vi "Shooter Controller.vi"(8 "error in":errorcluster) -> ()   [LabVIEW 2019]
doc: "This VI executes continuously carrying out the current operation and responding to updates or new operations. It will often contain the timing or control code that is difficult to place directly in TeleOp. This VI generally opens all sensors and motors and isolates the rest of the robot code from knowing how the operations are carried out."
uses:
  <vilib>/Rock Robotics/WPI/Framework/Completion Status.ctl
  Shooter Setpoints.ctl
  Shooter Operations.ctl
  <vilib>/Rock Robotics/WPI/MotorControl/WPI_MotorControlDeviceRef.ctl
  <vilib>/Rock Robotics/WPI/MotorControl/WPI_MotorControlType.ctl
  <vilib>/Rock Robotics/SystemInterfaces/DIO/FPGA_DIOPWMChannel.ctl
  <vilib>/Rock Robotics/WPI/PWM/WPI_PWMDeadband.ctl
  <vilib>/Rock Robotics/SystemInterfaces/DIO/FPGA_DIOChannel.ctl
  <vilib>/Rock Robotics/WPI/PWM/Servo/WPI_ServoDeviceRef.ctl
  <vilib>/Rock Robotics/WPI/ThirdParty/REV Robotics/SPARK MAX/Typedef/Spark MAX Motor Type.ctl
  <vilib>/Rock Robotics/WPI/ThirdParty/REV Robotics/SPARK MAX/Typedef/Spark MAX Control Type.ctl
panel:
  in  "Ramp Limit Rate (S)":sgl
  out "Shooter":T1(graph)
  in  "PID Shooter":T2={"P Gain"=0.00026, "I Gain"=0.0, "D Gain"=0.0, "F Gain"=0.0002, "I Zone"=0.0, "Min Output"=-1.0, "Max Output"=0.0} {"Max Output" min=-1.0 max=1.0 step=0.01; "Min Output" min=-1.0 max=1.0 step=0.01; "I Zone" step=0.01; "F Gain" step=0.01; "D Gain" step=0.01; "I Gain" step=0.01; "P Gain" min=0.0 step=0.01}
  in  "Interactive Values":T3
  out "Current\nCmd":string
  in  "Buttons":cluster{"Execute Cmd":bool, "Abort Cmd":bool}
  out "Command Timing":cluster{"Start Time (ms)":u32, "Iterations":i32}
  out "Status":T5
  # "Click here to set max"
  # "Click here to set min"
  # "Interactive Command: You may fill in the settings for a command\nand schedule it with the Execute button. You can observe and abort\nany command while fine tuning the code for the controller."
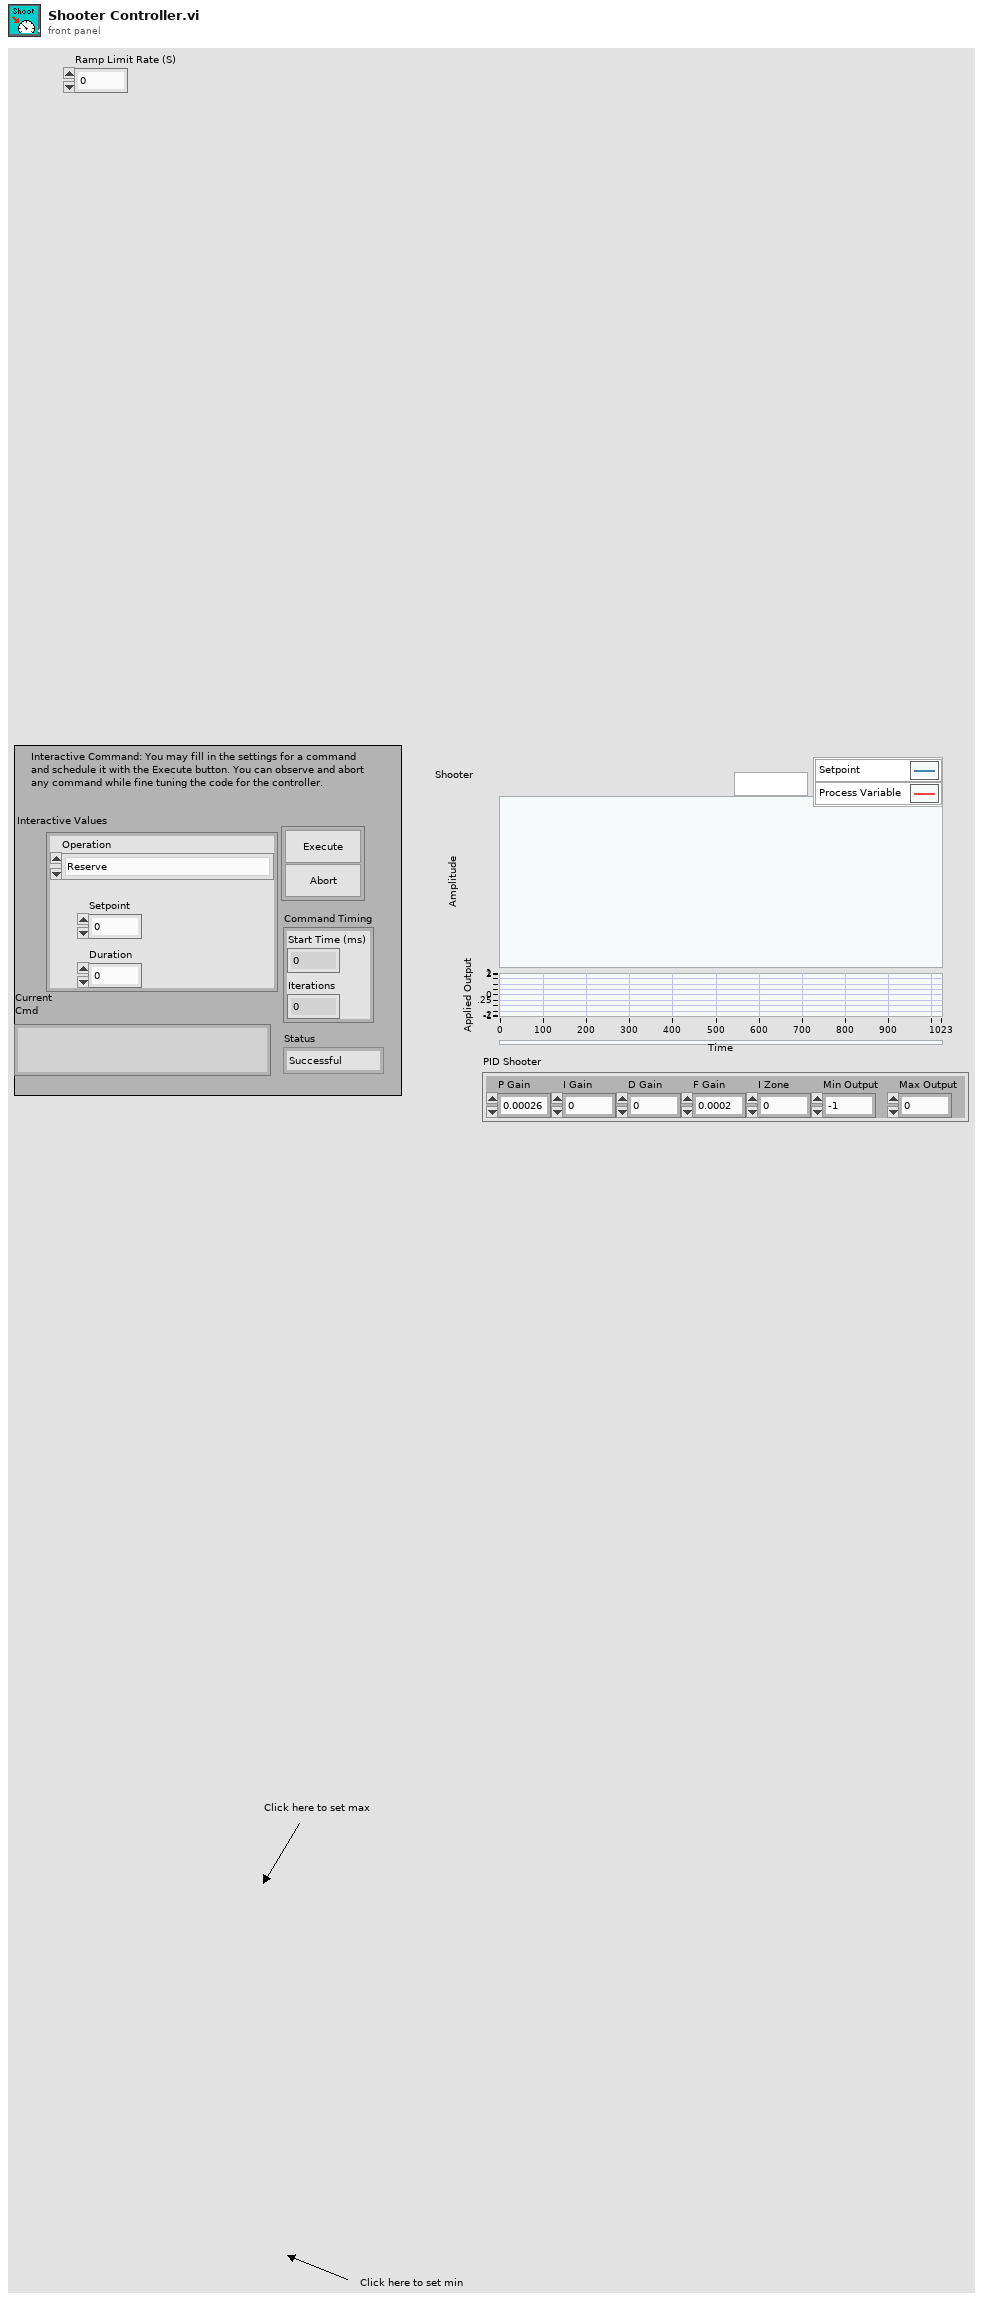
[diagram p1: front panel]
types:
  T1 = cluster{"Sensor Velocity":dbl, "Setpoint":dbl, "Applied Output":dbl}
  T2 = cluster{"P Gain":dbl, "I Gain":dbl, "D Gain":dbl, "F Gain":dbl, "I Zone":dbl, "Min Output":dbl, "Max Output":dbl}
  T3 = typedef "Shooter Setpoints.ctl" = cluster{"Operation":T4, "Setpoint":dbl, "Duration":dbl}
  T4 = typedef "Shooter Operations.ctl" = enum16{"Reserve", "Read Current", "Immediate", "Uptake", "Shooter", "Shift Winch", "Shift Uptake", "Shift Uptake Assist Up", "Shift Uptake Assist Down"}
  T5 = typedef "Completion Status.ctl" = enum16{"Successful", "Aborted", "Incomplete"}
  T6 = typedef "FPGA_DIOPWMChannel.ctl" = enum8{"PWM 0", "PWM 1", "PWM 2", "PWM 3", "PWM 4", "PWM 5", "PWM 6", "PWM 7", "PWM 8", "PWM 9", "PWM MXP 0", "PWM MXP 1", "PWM MXP 2", "PWM MXP 3", "PWM MXP 4", "PWM MXP 5", "PWM MXP 6", "PWM MXP 7", "PWM MXP 8", "PWM MXP 9", "Invalid"}
  T7 = typedef "Spark MAX Motor Type.ctl" = enum16{"Brushed", "Brushless"}
  T8 = typedef "WPI_MotorControlDeviceRef.ctl" = cluster{"DeviceStatus":errorcluster, "Type":T9, "PWM":cluster{"PWM Channel":T6, "DeadBand":T10}, "CAN":cluster{"Device Number":u8, "SetOutput VI Ref":variant, "GetOutput VI Ref":variant, "Enable VI Ref":variant, "Disable VI Ref":variant, "Data":variant}, "Invert":bool, "DIO PWM":cluster{"PWM \"Enable\" Channel":T6, "DIOChannel":T11, "PWM Rate":dbl}}
  T9 = typedef "WPI_MotorControlType.ctl" = enum16{"PWM", "CAN", "DIO PWM"}
  T10 = typedef "WPI_PWMDeadband.ctl" = cluster{"Name":string, "maxPositivePwm":i32, "minPositivePwm":i32, "centerPwm":i32, "maxNegativePwm":i32, "minNegativePwm":i32, "angularRange":u16}
  T11 = typedef "FPGA_DIOChannel.ctl" = enum8{"DIO 0", "DIO 1", "DIO 2", "DIO 3", "DIO 4", "DIO 5", "DIO 6", "DIO 7", "DIO 8", "DIO 9", "DIO MXP 0", "DIO MXP 1", "DIO MXP 2", "DIO MXP 3", "DIO MXP 4", "DIO MXP 5", "DIO MXP 6", "DIO MXP 7", "DIO MXP 8", "DIO MXP 9", "DIO MXP 10", "DIO MXP 11", "DIO MXP 12", "DIO MXP 13", "DIO MXP 14", "DIO MXP 15", "SPI Port CS1", "SPI Port CS2", "SPI Port CS3", "SPI Port MISO", "SPI Port MOSI", "Invalid"}
  T12 = typedef "WPI_ServoDeviceRef.ctl" = cluster{"DeviceStatus":errorcluster, "PWM Channel":T6, "DeadBand":T10}
  T13 = cluster{"Leader":T8, " Uptake":T8, "Setpoint for Shooter":dbl, "Setpoint for Uptake":dbl, "Shifter":T12, "Uptake Shifter ":T12}
  T14 = typedef "Command Status Info.ctl" = cluster{"Name":string, "Status":T5, "notifier out":T15}
  T15 = typedef "Completion Notifier.ctl" = refnum<notifier>
  T16 = cluster{"Current Command":T3, "Command Timing":cluster{"Start Time (ms)":u32, "Iterations":i32}, "Command Arguments":cluster{"Command Info":T14, "Description":string, "Default Command":T3, "queue out":refnum<queue>, "Subsystem Name":string}}
  T17 = typedef "Spark MAX Control Type.ctl" = enum16{"Percent VBus", "Voltage", "Velocity", "Position", "Smart Motion", "Current", "Smart Velocity"}
  T18 = cluster{"Sensor Velocity":dbl, "Setpoint for Shooter":dbl, "Applied Output":dbl}
  T19 = cluster{"P Gain":bool, "I Gain":bool, "D Gain":bool, "F Gain":bool, "I Zone":bool, "Min Output":bool, "Max Output":bool}
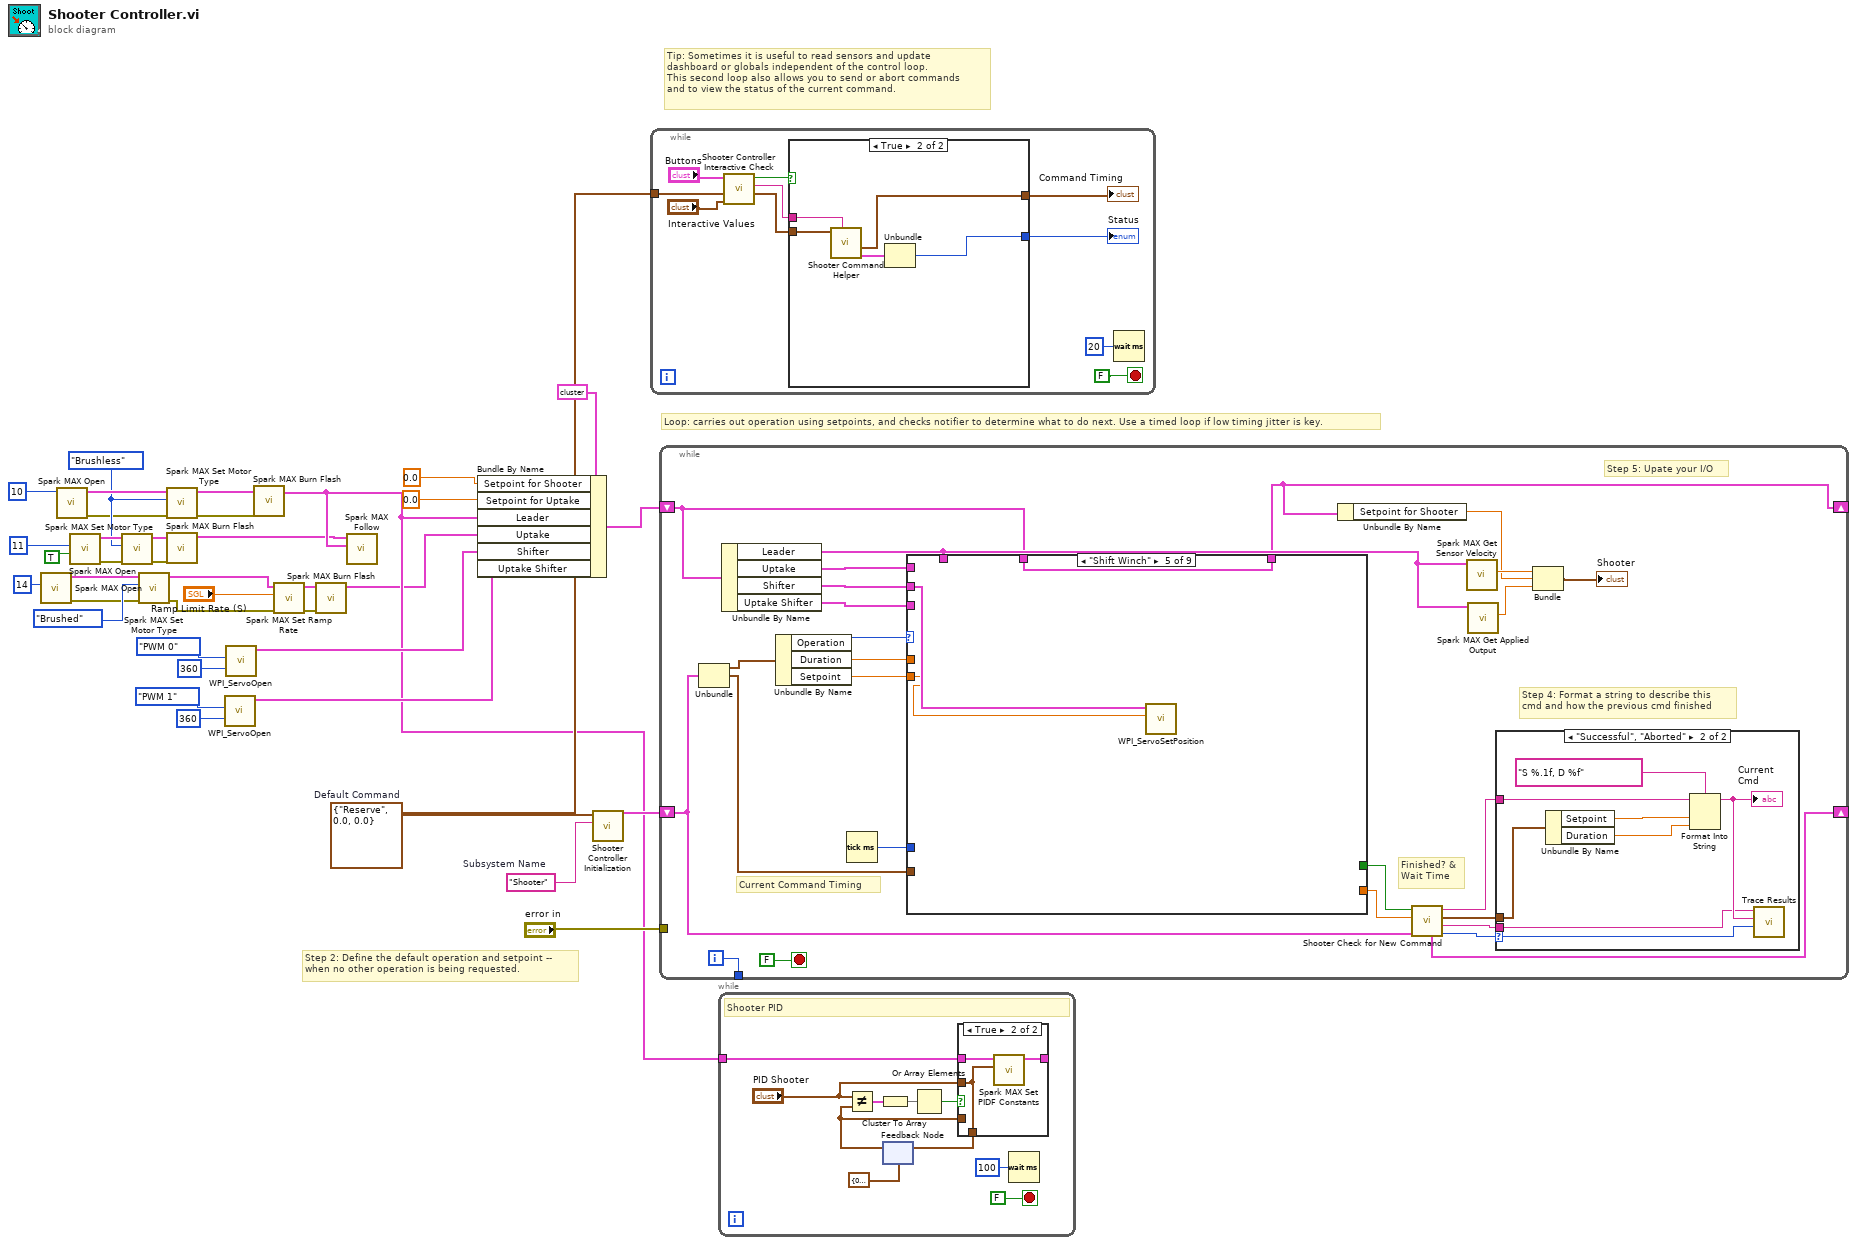
[diagram p0: block diagram]
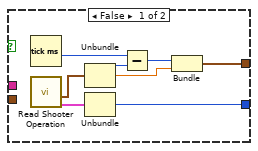
[diagram p2: hidden frame]
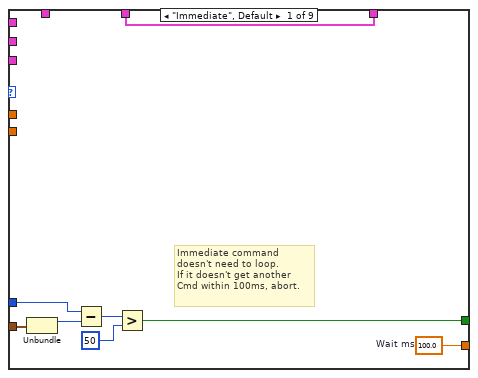
[diagram p5: hidden frame]
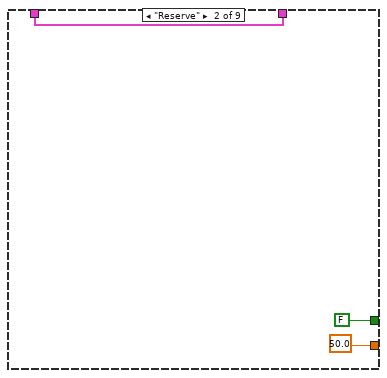
[diagram p6: hidden frame]
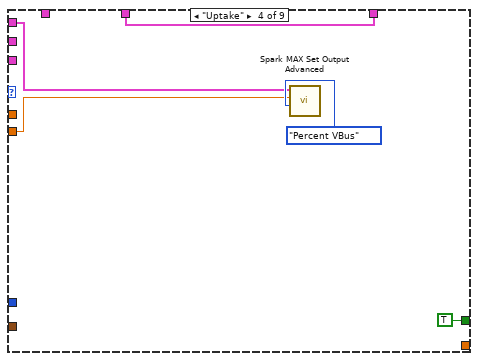
[diagram p8: hidden frame]
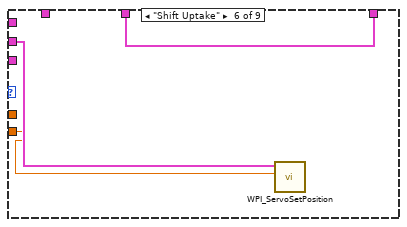
[diagram p9: hidden frame]
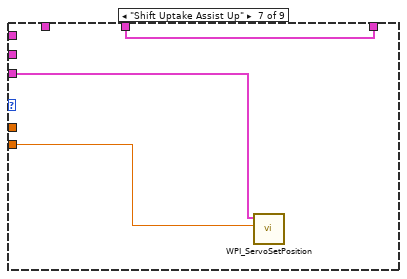
[diagram p10: hidden frame]
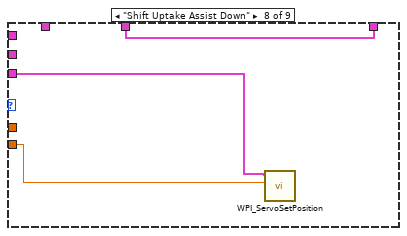
[diagram p11: hidden frame]
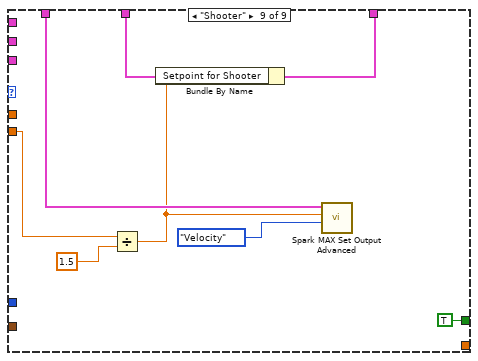
[diagram p12: hidden frame]
diagram:
  w22 = Spark_MAX_Motor_Type."Brushless" ("Motor Type")
  w35 = T3 {"Operation"=enum."Reserve", "Setpoint"=0.0, "Duration"=0.0}  # Default Command
  w36 = "Shooter"  # Subsystem Name
  # "Tip: Sometimes it is useful to read sensors and update\ndashboard or globals independent of the control loop.\nThis second loop also allows you to send or abort commands\nand to view the status of the current command."
  # "Step 2: Define the default operation and setpoint --\nwhen no other operation is being requested."
  # "Loop: carries out operation using setpoints, and checks notifier to determine what to do next. Use a timed loop if low timing jitter is key."
  n1 = call <vilib>:"Spark MAX Open.vi"("Device Number"=u8 14) -> ("error out"=w7:errorcluster, "MotorControlDeviceRef"=w29:T8)  [unwired: 9 in]
  n2 = call <vilib>:"Spark MAX Open.vi"("Device Number"=u8 10) -> ("error out"=w9:errorcluster, "MotorControlDeviceRef"=w23:T8)  [unwired: 9 in]
  n3 = call <vilib>:"Spark MAX Open.vi"("Invert"=TRUE, "Device Number"=u8 11) -> ("error out"=w8:errorcluster, "MotorControlDeviceRef"=w26:T8)  [unwired: 8 in]
  n4 = call <vilib>:"Spark MAX Set Motor Type.vi"("error in (no error)"=w8, "Motor Type"=w22, "MotorControlDevRef"=w26) -> ("error out"=w11:errorcluster, "MotorControlDeviceRef"=w12:T8)  [unwired: 7 in]
  n5 = call <vilib>:"Spark MAX Set Motor Type.vi"("error in (no error)"=w7, "Motor Type"=Spark_MAX_Motor_Type."Brushed", "MotorControlDevRef"=w29) -> ("error out"=w2:errorcluster, "MotorControlDeviceRef"=w5:T8)  [unwired: 7 in]
  n6 = call <vilib>:"Spark MAX Set Motor Type.vi"("error in (no error)"=w9, "Motor Type"=w22, "MotorControlDevRef"=w23) -> ("error out"=w15:errorcluster, "MotorControlDeviceRef"=w14:T8)  [unwired: 7 in]
  n7 = call <vilib>:"Spark MAX Burn Flash.vi"("error in"=w11, "MotorControlDeviceRef"=w12) -> ("MotorControlDeviceRef"=w6:T8)  [unwired: 8 in, 1 out]
  n8 = call <vilib>:"WPI_ServoOpen.vi"("Angular Range"=u16 360, "PWM Channel"=FPGA_DIOPWMChannel."PWM 1") -> ("ServoDeviceRef"=w16:T12)  [unwired: 8 in, 1 out]
  n9 = call <vilib>:"WPI_ServoOpen.vi"("Angular Range"=u16 360, "PWM Channel"=FPGA_DIOPWMChannel."PWM 0") -> ("ServoDeviceRef"=w21:T12)  [unwired: 8 in, 1 out]
  n10 = call <vilib>:"Spark MAX Burn Flash.vi"("error in"=w15, "MotorControlDeviceRef"=w14) -> ("MotorControlDeviceRef"=w13:T8)  [unwired: 8 in, 1 out]
  n11 = call <vilib>:"Spark MAX Set Ramp Rate.vi"("error in (no error)"=w2, "Seconds from neutral to full (0)"="Ramp Limit Rate (S)", "MotorControlDeviceRef in"=w5) -> ("error out"=w3:errorcluster, "MotorControlDeviceRef"=w4:T8)  [unwired: 7 in]
  n12 = call <vilib>:"Spark MAX Burn Flash.vi"("error in"=w3, "MotorControlDeviceRef"=w4) -> ("MotorControlDeviceRef"=w10:T8)  [unwired: 8 in, 1 out]
  n13 = call <vilib>:"Spark MAX Follow.vi"("Master Controller"=w13, "MotorControlDeviceRef"=w6) -> ()  [unwired: 8 in, 2 out]
  n14 = Bundle By Name(cluster=T13 {"Leader"={"DeviceStatus"={"status"=FALSE, "code"=0, "source"=""}, "Type"=enum."PWM", "PWM"={"PWM Channel"=enum."Invalid", "DeadBand"={"Name"="", "maxPositivePwm"=0, "minPositivePwm"=0, "centerPwm"=0, "maxNegativePwm"=0, "minNegativePwm"=0, "angularRange"=0}}, "CAN"={"Device Number"=0, "SetOutput VI Ref"=variant(refnum<vi> refnum), "GetOutput VI Ref"=variant(refnum<vi> refnum), "Enable VI Ref"=variant(refnum<vi> refnum), "Disable VI Ref"=variant(refnum<vi> refnum), "Data"=variant}, "Invert"=FALSE, "DIO PWM"={"PWM \"Enable\" Channel"=enum."Invalid", "DIOChannel"=enum."Invalid", "PWM Rate"=0.0}}, " Uptake"={"DeviceStatus"={"status"=FALSE, "code"=0, "source"=""}, "Type"=enum."PWM", "PWM"={"PWM Channel"=enum."Invalid", "DeadBand"={"Name"="", "maxPositivePwm"=0, "minPositivePwm"=0, "centerPwm"=0, "maxNegativePwm"=0, "minNegativePwm"=0, "angularRange"=0}}, "CAN"={"Device Number"=0, "SetOutput VI Ref"=variant(refnum<vi> refnum), "GetOutput VI Ref"=variant(refnum<vi> refnum), "Enable VI Ref"=variant(refnum<vi> refnum), "Disable VI Ref"=variant(refnum<vi> refnum), "Data"=variant}, "Invert"=FALSE, "DIO PWM"={"PWM \"Enable\" Channel"=enum."Invalid", "DIOChannel"=enum."Invalid", "PWM Rate"=0.0}}, "Setpoint for Shooter"=0.0, "Setpoint for Uptake"=0.0, "Shifter"={"DeviceStatus"={"status"=FALSE, "code"=0, "source"=""}, "PWM Channel"=enum."Invalid", "DeadBand"={"Name"="", "maxPositivePwm"=0, "minPositivePwm"=0, "centerPwm"=0, "maxNegativePwm"=0, "minNegativePwm"=0, "angularRange"=0}}, "Uptake Shifter "={"DeviceStatus"={"status"=FALSE, "code"=0, "source"=""}, "PWM Channel"=enum."Invalid", "DeadBand"={"Name"="", "maxPositivePwm"=0, "minPositivePwm"=0, "centerPwm"=0, "maxNegativePwm"=0, "minNegativePwm"=0, "angularRange"=0}}} ("output cluster"), "Setpoint for Shooter"=0.0 ("Shooter Setpoint"), "Setpoint for Uptake"=0.0 ("Uptake Setpoint"), "Leader"=w13, "Uptake"=w10, "Shifter"=w21, "Uptake Shifter"=w16) -> (w28:T13)
  n15 = call "Shooter Controller Initialization.vi"("Subsystem Name"=w36, "Default Command"=w35) -> ("Current Command"=w37:T16)  [unwired: 9 in]
  n16 = while {
    tunnel: w35 -> [w45]
    stop <- FALSE stop-if-true
    n17 = call "Shooter Controller Interactive Check.vi"("Interactive Command in"="Interactive Values", "Default Command"=w45, "Buttons"="Buttons") -> ("Interactive Command out"=w42:T3, "Trace String"=w43:string, "Schedule"=w44:bool)  [unwired: 6 in]
    n18 = case shown="True" w44 {
      tunnel: [w56 w61] -> w41
      tunnel: w42 -> [_ w59]
      tunnel: [w52 w57] -> w40
      tunnel: w43 -> [_ w60]
      frame False {
        n19 = Tick Count (ms)() -> (millisecond timer value=w51:u32)
        n20 = call "Read Shooter Operation.vi"() -> ("Command Info"=w49:T14, "SubSystem Data"=w50:T3)  [unwired: 9 in, 1 out]
        n21 = Unbundle(w50) -> ("Operation"=w55:T4, "Setpoint"=w53:dbl)  [unwired: 1 out]
        n22 = Unbundle(w49) -> ("Status"=w56:T5)  [unwired: 2 out]
        n23 = Subtract(x=w51, y=w55) -> (x-y=w54:u32)
        n24 = Bundle(w54, "Setpoint"=w53) -> (w52:cluster{u32, "Setpoint":dbl})  [unwired: 1 in]
      }
      frame True {
        n25 = call "Shooter Command Helper.vi"("Description"=w60, "SubSystem Data"=w59) -> ("Command Info Out"=w58:T14, "Command Timing"=w57:cluster{"Start Time (ms)":u32, "Iterations":i32})  [unwired: 7 in, 1 out]
        n26 = Unbundle(w58) -> ("Status"=w61:T5)  [unwired: 2 out]
      }
    }
    "Status" <- w41
    "Command Timing" <- w40
    n27 = Wait (ms)(milliseconds to wait=u32 20) -> ()  [unwired: 1 out]
  }
  n28 = while {
    shift-right: [w79] -> _
    shift-left: w37 -> [w72]
    tunnel: [w86] -> _
    tunnel: "error in" -> [_]
    shift-right: [w65] -> _
    shift-left: w28 -> [w66]
    i -> [w86]
    stop <- FALSE stop-if-true
    # "Step 5: Upate your I/O"
    # "Step 4: Format a string to describe this\ncmd and how the previous cmd finished"
    # "Current Command Timing"
    # "Finished? &\nWait Time"
    n29 = Unbundle(w72) -> ("Current Command"=w85:T3, "Command Timing"=w81:cluster{"Start Time (ms)":u32, "Iterations":i32})  [unwired: 1 out]
    n30 = Unbundle By Name(w66) -> ("Leader"=w71:T8, "Uptake"=w70:T8, "Shifter"=w63:T12, "Uptake Shifter"=w62:T12)
    n31 = Unbundle By Name(w85) -> ("Operation"=w84:T4, "Duration"=w83:dbl, "Setpoint"=w80:dbl)
    n32 = Tick Count (ms)() -> (millisecond timer value=w82:u32)
    n33 = case shown="\"Shift Winch\"" w84 {
      tunnel: [w103 50.0 _ _ _ _ _ _ _] -> w77
      tunnel: [w97 FALSE ("ignore previous (F)") _ TRUE ("ignore previous (F)") _ _ _ _ TRUE ("ignore previous (F)")] -> w78
      tunnel: w81 -> [w99 _ _ _ _ _ _ _ _]
      tunnel: w83 -> [_ _ _ _ _ _ _ _ _]
      tunnel: w82 -> [w98 _ _ _ _ _ _ _ _]
      tunnel: w80 -> [_ _ _ w109 w113 w116 w119 w122 w129]
      tunnel: w71 -> [_ _ _ _ _ _ _ _ w131]
      tunnel: w70 -> [_ _ _ w108 _ _ _ _ _]
      tunnel: w66 -> [w96 w104 w107 w111 w115 w118 w121 w124 w127]
      tunnel: [w96 w104 w107 w111 w115 w118 w121 w124 w125] -> w65
      tunnel: w63 -> [_ _ _ _ w114 w117 _ _ _]
      tunnel: w62 -> [_ _ _ _ _ _ w120 w123 _]
      frame "Immediate", Default {
        w103 = 100.0  # Wait ms
        # "Immediate command\ndoesn't need to loop.\nIf it doesn't get another\nCmd within 100ms, abort."
        n34 = Unbundle(w99) -> ("Start Time (ms)"=w102:u32)  [unwired: 1 out]
        n35 = Subtract(x=w98, y=w102) -> (x-y=w101:u32)
        n36 = Greater?(x=w101, y=u8 50 ("Left Motor")) -> (0:w97:bool)
      }
      frame "Reserve" {
      }
      frame "Read Current" {
      }
      frame "Uptake" {
        n37 = call <vilib>:"Spark MAX Set Output Advanced.vi"("Control Mode"=Spark_MAX_Control_Type."Percent VBus", "Setpoint"=w109, "MotorControlDevRef"=w108) -> ()  [unwired: 7 in, 2 out]
      }
      frame "Shift Winch" {
        n38 = call <vilib>:"WPI_ServoSetPosition.vi"("Position"=w113, "ServoDeviceRef"=w114) -> ()  [unwired: 8 in, 2 out]
      }
      frame "Shift Uptake" {
        n39 = call <vilib>:"WPI_ServoSetPosition.vi"("Position"=w116, "ServoDeviceRef"=w117) -> ()  [unwired: 8 in, 2 out]
      }
      frame "Shift Uptake Assist Up" {
        n40 = call <vilib>:"WPI_ServoSetPosition.vi"("Position"=w119, "ServoDeviceRef"=w120) -> ()  [unwired: 8 in, 2 out]
      }
      frame "Shift Uptake Assist Down" {
        n41 = call <vilib>:"WPI_ServoSetPosition.vi"("Position"=w122, "ServoDeviceRef"=w123) -> ()  [unwired: 8 in, 2 out]
      }
      frame "Shooter" {
        n42 = Divide(x=w129, y=1.5) -> (x/y=w126:dbl)
        n43 = Bundle By Name(cluster=w127, "Setpoint for Shooter"=w126) -> (w125:T13)
        n44 = call <vilib>:"Spark MAX Set Output Advanced.vi"("Control Mode"=Spark_MAX_Control_Type."Velocity", "Setpoint"=w126, "MotorControlDevRef"=w131) -> ()  [unwired: 7 in, 2 out]
      }
    }
    n45 = Unbundle By Name(w65) -> ("Setpoint for Shooter"=w64:dbl)
    n46 = call "Shooter Check for New Command.vi"("Current Command"=w72, "Wait time (ms)"=w77, "Finished?"=w78) -> ("Completion"=w73:T5, "Subsystem Name"=w74:string, "Current Command"=w75:T3, "Initial Trace String"=w76:string, "NextCommand"=w79:T16)  [unwired: 4 in]
    n47 = call <vilib>:"Spark MAX Get Sensor Velocity.vi"("MotorControlDevRef in"=w71) -> ("Sensor Velocity"=w68:dbl)  [unwired: 7 in, 3 out]
    n48 = call <vilib>:"Spark MAX Get Applied Output.vi"("MotorControlDevRef in"=w71) -> ("Applied Output"=w69:dbl)  [unwired: 7 in, 3 out]
    n49 = case shown="\"Successful\", \"Aborted\"" w73 {
      selector: w73 -> [_ w95]
      tunnel: w76 -> [_ w91]
      tunnel: w75 -> [_ w92]
      tunnel: w74 -> [_ w88]
      frame "Incomplete", Default {
        # "Continuing current command"
      }
      frame "Successful", "Aborted" {
        # "Report and setup for next command"
        n50 = Unbundle By Name(w92) -> ("Setpoint"=w94:dbl, "Duration"=w89:dbl)
        n51 = Format Into String(format string="S %.1f, D %f", initial string=w91, w94, w89) -> (resulting string=w90:string)  [unwired: 1 in, 1 out]
        "Current\nCmd" <- w90
        n52 = call <vilib>:"Trace Results.vi"("Status of previous command"=w95, "Description"=w90, "Subsystem"=w88) -> ()  [unwired: 9 in]
      }
    }
    n53 = Bundle("Sensor Velocity"=w68, "Setpoint for Shooter"=w64, "Applied Output"=w69) -> (→"Shooter":T18)  [unwired: 1 in]
  }
  n54 = while {
    tunnel: w13 -> [w133]
    stop <- FALSE stop-if-true
    # "Shooter PID"
    n55 = feedback #1(T2 {"P Gain"=0.0, "I Gain"=0.0, "D Gain"=0.0, "F Gain"=0.0, "I Zone"=0.0, "Min Output"=0.0, "Max Output"=0.0} ("PID Constants")) -> (w142:T2)
    n56 = Not Equal?(x="PID Shooter", y=w142) -> (x != y?=w136:T19)
    n57 = Cluster To Array(cluster=w136) -> (array=w137:bool[])
    n58 = Or Array Elements(Boolean array=w137) -> (logical OR=w139:bool)
    n59 = case shown="True" w139 {
      tunnel: "PID Shooter" -> [_ w145]
      tunnel: [w143 w145] -> w141
      tunnel: w142 -> [w143 _]
      tunnel: [_ w146] -> _
      tunnel: w133 -> [_ w144]
      frame False {
      }
      frame True {
        n60 = call <vilib>:"Spark MAX Set PIDF Constants.vi"("PID Constants"=w145, "MotorControlDeviceRef"=w144) -> ("MotorControlDeviceRef"=w146:T8)  [unwired: 8 in, 1 out]
      }
    }
    n61 = feedback-in #1(w141) -> ()
    n62 = Wait (ms)(milliseconds to wait=u32 100) -> ()  [unwired: 1 out]
  }
